vi "Empty string is an Object.vi"(11 "JSON Input":string) -> (3 "<JSON>Object":string)   [LabVIEW 2020, in "JSONtext.lvlib"]
uses:
  <vilib>/JDP Science/JSONtext/JSONtext.lvlib
panel:
  # "Make empty input count as {}"
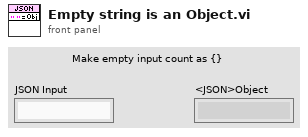
[diagram p1: front panel]
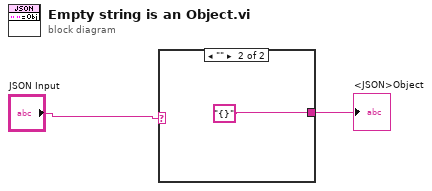
[diagram p0: block diagram]
diagram:
  n1 = case shown="\"\"" "JSON Input" {
    selector: "JSON Input" -> [w3 _]
    tunnel: [w3 "{}"] -> w2
    frame Default {
    }
    frame "" {
    }
  }
  "<JSON>Object" <- w2
